vi "ReportPart.vi"(6 "试验项目":T2(ring), 8 "error in":errorcluster, 9 "索引IN":i32, 10 "合格":T1, 11 "report in":refnum<class "NI_report.lvclass">) -> (0 "error out 2":errorcluster caption="error out", 2 "索引OUT":i32, 3 "report out":refnum<class "NI_report.lvclass">)   [LabVIEW 2020]
uses:
  <vilib>/Utility/NIReport.llb/NI_report.lvclass
  OK.ctl
  <vilib>/Utility/NIReport.llb/image depth.ctl
  <vilib>/addons/_office/_exclsub.llb/font.ctl
  Global_Variable/A180648.vi
  <vilib>/Utility/NIReport.llb/Append Report Text (str wrap).vi
  Global_Variable/Global.vi
  <vilib>/addons/_office/word.llb/Word Easy Table (str).vi
  <vilib>/Utility/NIReport.llb/NI_ReportGenerationCore.lvlib
  <vilib>/addons/_office/NI_ReportGenerationToolkit.lvlib
  <vilib>/Utility/NIReport.llb/Word/NI_Word.lvclass
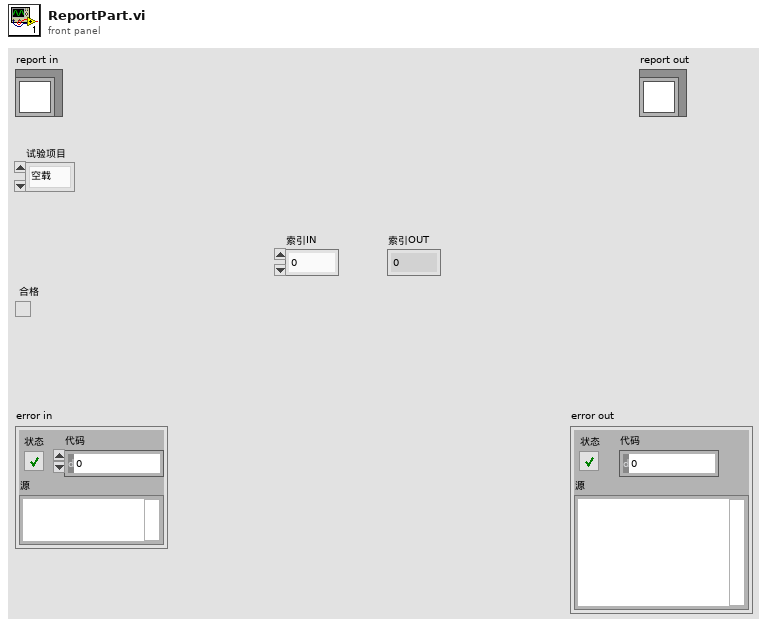
[diagram p1: front panel]
types:
  T1 = typedef "OK.ctl" = bool
  T2 = enum32{"空载", "功能", "力特性", "电流特性", "传感器特性", "逆向空载", "振动NVH", "磨合"}
  T3 = cluster{"Charset (-1)":i16, "Weight (-1)":i16, "Name":string, "Size":string}
  T4 = cluster{"Italic":enum16{"Italic Unchanged", "Italic On", "Italic Off"}, "Strike Through":enum16{"Strike Through Unchanged", "Strike Through On", "Strike Through Off"}, "Underline":enum16{"Underline Unchanged", "Underline On", "Underline Off"}, "Bold":enum16{"Bold Unchanged", "Bold On", "Bold Off"}}
  T5 = typedef "NI_ReportGenerationToolkit.lvlib/font.ctl" = cluster{"font name":string, "font size":dbl, "bold":u16, "italic":u16, "underline":u16, "strike through":u16, "font color":u32}
  T6 = typedef "NI_ReportGenerationCore.lvlib/image depth.ctl" = u16
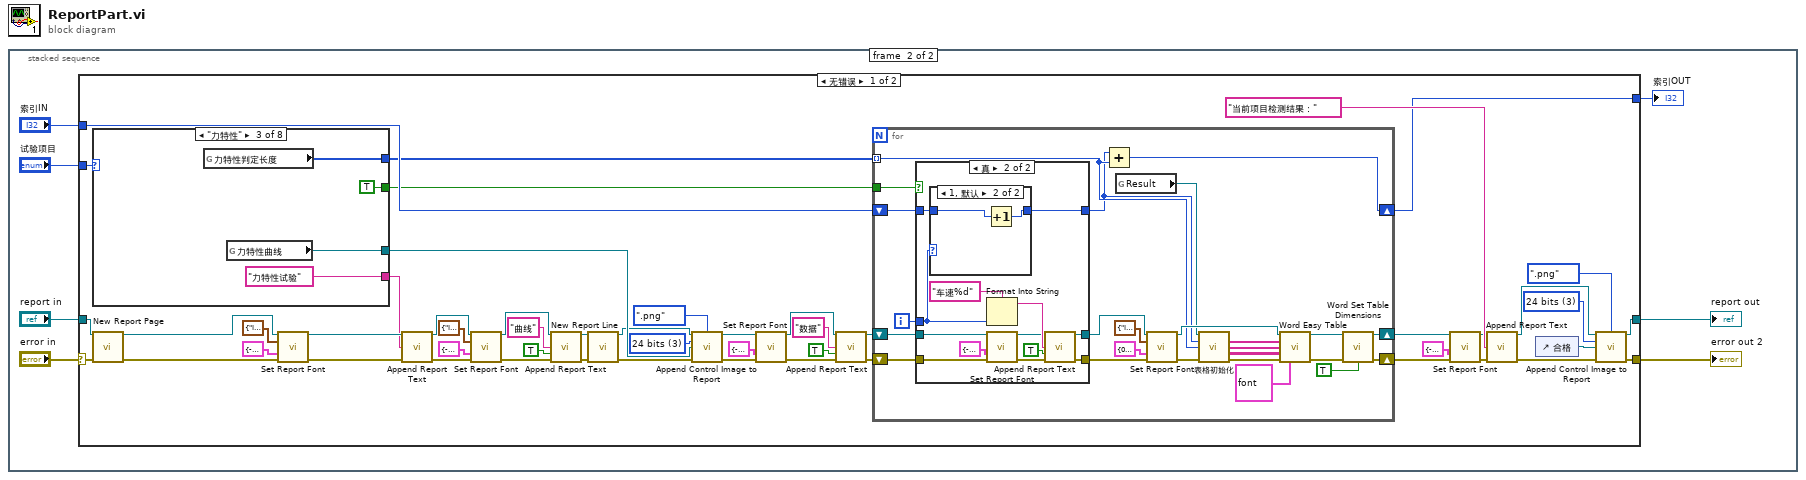
[diagram p0: block diagram]
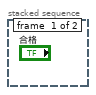
[diagram p2: hidden frame]
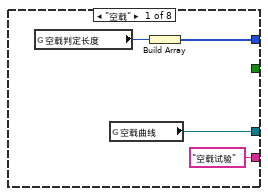
[diagram p5: hidden frame]
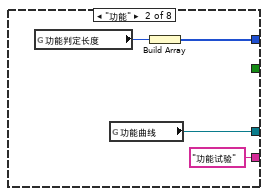
[diagram p6: hidden frame]
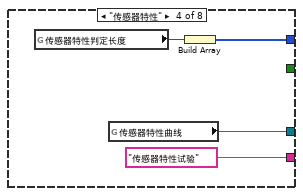
[diagram p7: hidden frame]
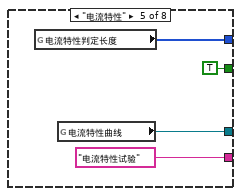
[diagram p8: hidden frame]
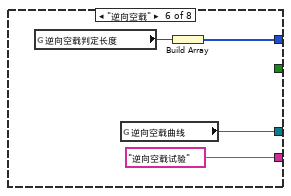
[diagram p9: hidden frame]
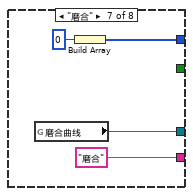
[diagram p10: hidden frame]
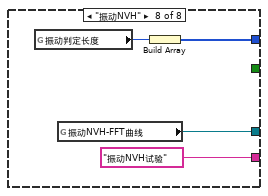
[diagram p11: hidden frame]
diagram:
  n1 = stacked-sequence {
    frame #0 {
    }
    frame #1 {
      n2 = case shown="无错误" "error in" {
        selector: "error in" -> [w51 w137]
        tunnel: [w46 w137] -> w6
        tunnel: "索引IN" -> [w18 w136]
        tunnel: "试验项目" -> [w21 _]
        tunnel: [w15 w136] -> w3
        tunnel: [w20 w135] -> w2
        tunnel: "report in" -> [w19 w135]
        frame No Error {
          w34 = T6 3 items=["B&W", "4 bits", "8 bits", "24 bits"] ("image depth")
          w44 = T6 3 items=["B&W", "4 bits", "8 bits", "24 bits"] ("image depth")
          n3 = case shown="\"力特性\"" w21 {
            tunnel: [w106 w110 w114 w117 w122 w125 w129 w133] -> w37
            tunnel: ["空载试验" ("text") "功能试验" ("text") "力特性试验" ("text") "传感器特性试验" ("text") "电流特性试验" ("text") "逆向空载试验" ("text") "磨合" ("text") "振动NVH试验" ("text")] -> w55
            tunnel: [w103 w107 w112 w115 w120 w123 w128 w131] -> w17
            tunnel: [_ _ TRUE _ TRUE _ _ _] -> w14
            frame "空载" {
              n4 = global read "判定参数.vi" "空载判定长度"() -> (w104:i32)
              n5 = global read "A180648.vi" "空载曲线"() -> (w106:refnum<vi>)
              n6 = Build Array(w104) -> (w103:i32[])
            }
            frame "功能" {
              n7 = global read "判定参数.vi" "功能判定长度"() -> (w108:i32)
              n8 = global read "A180648.vi" "功能曲线"() -> (w110:refnum<vi>)
              n9 = Build Array(w108) -> (w107:i32[])
            }
            frame "力特性" {
              n10 = global read "判定参数.vi" "力特性判定长度"() -> (w112:i32[])
              n11 = global read "A180648.vi" "力特性曲线"() -> (w114:refnum<vi>)
            }
            frame "传感器特性" {
              n12 = global read "判定参数.vi" "传感器特性判定长度"() -> (w116:i32)
              n13 = global read "A180648.vi" "传感器特性曲线"() -> (w117:refnum<vi>)
              n14 = Build Array(w116) -> (w115:i32[])
            }
            frame "电流特性" {
              n15 = global read "判定参数.vi" "电流特性判定长度"() -> (w120:i32[])
              n16 = global read "A180648.vi" "电流特性曲线"() -> (w122:refnum<vi>)
            }
            frame "逆向空载" {
              n17 = global read "判定参数.vi" "逆向空载判定长度"() -> (w124:i32)
              n18 = global read "A180648.vi" "逆向空载曲线"() -> (w125:refnum<vi>)
              n19 = Build Array(w124) -> (w123:i32[])
            }
            frame "磨合" {
              n20 = global read "A180648.vi" "磨合曲线"() -> (w129:refnum<vi>)
              n21 = Build Array(0 ("元素")) -> (w128:i32[])
            }
            frame "振动NVH" {
              n22 = global read "判定参数.vi" "振动判定长度"() -> (w132:i32)
              n23 = global read "A180648.vi" "振动NVH-FFT曲线"() -> (w133:refnum<vi>)
              n24 = Build Array(w132) -> (w131:i32[])
            }
          }
          n25 = call-dynamic "New Report Page.vi"("report in"=w19, "error in (no error)"=w51) -> ("report out"=w49:refnum<class "NI_report.lvclass">, "error out"=w50:errorcluster)  [unwired: 12 in]
          n26 = call-dynamic "Set Report Font.vi"("report in"=w49, "text options"=T4 {"Italic"=enum."Italic Unchanged", "Strike Through"=enum."Strike Through Unchanged", "Underline"=enum."Underline Unchanged", "Bold"=enum."Bold On"}, "font settings"=T3 {"Charset (-1)"=-1, "Weight (-1)"=-1, "Name"="楷体", "Size"="16 "}, "error in (no error)"=w50) -> ("report out"=w58:refnum<class "NI_report.lvclass">, "error out"=w57:errorcluster)  [unwired: 9 in, 1 out]
          n27 = call-poly <vilib>:"Append Report Text.vi"("report in"=w58, "text"=w55, "error in (no error)"=w57) -> ("report out"=w53:refnum<class "NI_report.lvclass">, "error out"=w52:errorcluster)  [unwired: 9 in, 2 out]
          n28 = call-dynamic "Set Report Font.vi"("report in"=w53, "text options"=T4 {"Italic"=enum."Italic Unchanged", "Strike Through"=enum."Strike Through Unchanged", "Underline"=enum."Underline Unchanged", "Bold"=enum."Bold Off"}, "font settings"=T3 {"Charset (-1)"=-1, "Weight (-1)"=-1, "Name"="宋体", "Size"="12"}, "error in (no error)"=w52) -> ("report out"=w28:refnum<class "NI_report.lvclass">, "error out"=w25:errorcluster)  [unwired: 9 in, 1 out]
          n29 = call-poly <vilib>:"Append Report Text.vi"("report in"=w28, "text"="曲线", "append on new line? (F)"=TRUE, "error in (no error)"=w25) -> ("report out"=w27:refnum<class "NI_report.lvclass">, "error out"=w26:errorcluster)  [unwired: 8 in, 2 out]
          n30 = call-dynamic "New Report Line.vi"("report in"=w27, "error in (no error)"=w26) -> ("report out"=w35:refnum<class "NI_report.lvclass">, "error out"=w36:errorcluster)  [unwired: 12 in]
          n31 = call-dynamic "Append Control Image to Report.vi"("report in"=w35, "image file type (.jpg)"=enum16{".jpg", ".png"}.".png", "image depth"=w34, "ctrl reference"=w37, "error in (no error)"=w36) -> ("report out"=w32:refnum<class "NI_report.lvclass">, "error out"=w31:errorcluster)  [unwired: 7 in, 2 out]
          n32 = call-dynamic "Set Report Font.vi"("report in"=w32, "font settings"=T3 {"Charset (-1)"=-1, "Weight (-1)"=-1, "Name"="微软雅黑", "Size"="12 "}, "error in (no error)"=w31) -> ("report out"=w13:refnum<class "NI_report.lvclass">, "error out"=w10:errorcluster)  [unwired: 10 in, 1 out]
          n33 = call-poly <vilib>:"Append Report Text.vi"("report in"=w13, "text"="数据", "append on new line? (F)"=TRUE, "error in (no error)"=w10) -> ("report out"=w9:refnum<class "NI_report.lvclass">, "error out"=w8:errorcluster)  [unwired: 8 in, 2 out]
          n34 = for {
            tunnel: w17 -> [w68] mode=indexing
            shift-right: [w83] -> w39
            shift-left: w9 -> [w66]
            shift-right: [w82] -> w38
            shift-left: w8 -> [w65]
            shift-right: [w67] -> w15
            shift-left: w18 -> [w60]
            tunnel: w14 -> [w61]
            i -> [w62]
            n35 = case shown="真" w61 {
              tunnel: w66 -> [w86 w93]
              tunnel: w65 -> [w85 w92]
              tunnel: [w86 w91] -> w64
              tunnel: [w85 w90] -> w63
              tunnel: w62 -> [_ w87]
              tunnel: w60 -> [w84 w89]
              tunnel: [w84 w88] -> w59
              frame False {
              }
              frame True {
                n36 = case shown="1, 默认" w87 {
                  tunnel: [w100 w101] -> w88
                  tunnel: w89 -> [w100 w102]
                  frame 0 {
                  }
                  frame 1, Default {
                    n37 = Increment(x=w102) -> (x+1=w101:i32)
                  }
                }
                n38 = Format Into String(format string="车速%d" ("格式字符串"), w87) -> (resulting string=w99:string)  [unwired: 2 in, 1 out]
                n39 = call-dynamic "Set Report Font.vi"("report in"=w93, "font settings"=T3 {"Charset (-1)"=-1, "Weight (-1)"=-1, "Name"="宋体", "Size"="12 "}, "error in (no error)"=w92) -> ("report out"=w98:refnum<class "NI_report.lvclass">, "error out"=w97:errorcluster)  [unwired: 10 in, 1 out]
                n40 = call-poly <vilib>:"Append Report Text.vi"("report in"=w98, "text"=w99, "append on new line? (F)"=TRUE, "error in (no error)"=w97) -> ("report out"=w91:refnum<class "NI_report.lvclass">, "error out"=w90:errorcluster)  [unwired: 8 in, 2 out]
              }
            }
            n41 = Add(x=w59, y=w68) -> (x+y=w67:i32)
            n42 = global read "Global.vi" "Result"() -> (w69:refnum<vi>)
            n43 = call-dynamic "Set Report Font.vi"("report in"=w64, "text options"=T4 {"Italic"=enum."Italic Unchanged", "Strike Through"=enum."Strike Through Unchanged", "Underline"=enum."Underline Unchanged", "Bold"=enum."Bold Unchanged"}, "font settings"=T3 {"Charset (-1)"=0, "Weight (-1)"=-1, "Name"="微软雅黑", "Size"="12 "}, "error in (no error)"=w63) -> ("report out"=w71:refnum<class "NI_report.lvclass">, "error out"=w70:errorcluster)  [unwired: 9 in, 1 out]
            n44 = call "表格初始化.vi"("表格引用"=w69, "索引"=w59, "长度"=w68, "错误输入（无错误）"=w70) -> ("行首字符串[]"=w73:string[], "列首字符串[]"=w72:string[], "文本数据"=w75:string[][], "错误输出"=w78:errorcluster)  [unwired: 7 in, 1 out]
            n45 = call-poly <vilib>:"Word Easy Table.vi"("report in"=w71, "row headers"=w73, "column headers"=w72, "data"=w75, "error in (no error)"=w78, "font"=T5 {"font name"="宋体", "font size"=12.0, "bold"=2, "italic"=2, "underline"=2, "strike through"=2, "font color"=16777216}) -> ("report out"=w76:refnum<class "NI_report.lvclass">, "error out"=w77:errorcluster)  [unwired: 7 in, 1 out]
            n46 = call <vilib>:"Word Set Table Dimensions.vi"("report in"=w76, "error in (no error)"=w77, "fit to page width? (F)"=TRUE) -> ("report out"=w83:refnum<class "NI_report.lvclass">, "error out"=w82:errorcluster)  [unwired: 11 in]
          }
          n47 = call-dynamic "Set Report Font.vi"("report in"=w39, "font settings"=T3 {"Charset (-1)"=-1, "Weight (-1)"=-1, "Name"="宋体", "Size"="16 "}, "error in (no error)"=w38) -> ("report out"=w42:refnum<class "NI_report.lvclass">, "error out"=w43:errorcluster)  [unwired: 10 in, 1 out]
          n48 = call-poly <vilib>:"Append Report Text.vi"("report in"=w42, "text"="当前项目检测结果：", "error in (no error)"=w43) -> ("report out"=w48:refnum<class "NI_report.lvclass">, "error out"=w47:errorcluster)  [unwired: 9 in, 2 out]
          n49 = control-ref of="合格"() -> (w16:refnum<vi>)
          n50 = call-dynamic "Append Control Image to Report.vi"("report in"=w48, "image file type (.jpg)"=enum16{".jpg", ".png"}.".png", "image depth"=w44, "ctrl reference"=w16, "error in (no error)"=w47) -> ("report out"=w20:refnum<class "NI_report.lvclass">, "error out"=w46:errorcluster)  [unwired: 7 in, 2 out]
        }
        frame Error {
        }
      }
      "error out 2" <- w6
      "索引OUT" <- w3
      "report out" <- w2
    }
  }
